vi "read allowed execution modes.vi"(8 "error in":errorcluster, 11 "Modbus Slave editor node in":refnum<class "Modbus Slave editor node.lvclass">) -> (0 "error out":errorcluster, 2 "allowed execution modes":T1[](array[typedef]), 3 "Modbus Slave editor node out":refnum<class "Modbus Slave editor node.lvclass">)   [LabVIEW 2013, in "Modbus Slave editor node.lvclass"]
doc: "Platypus Framework 1.0.1.65\nNI Systems Engineering - National Instruments"
uses:
  Modbus Slave editor node.lvclass
  <vilib>/NI/Tag Bus Data Framework/Configuration Editor/Classes/Module editor node/Allowed Execution Modes.ctl
  <vilib>/NI/Tag Bus Data Framework/Configuration Editor/Classes/Module editor node/module editor node.lvclass
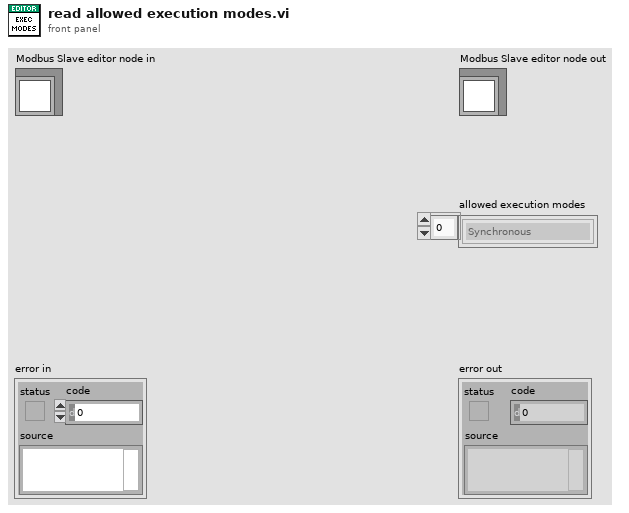
[diagram p1: front panel]
types:
  T1 = typedef "PL Framework Configuration Tool.lvlib/module editor node.lvclass/Allowed Execution Modes.ctl" = enum16{"Synchronous", "Asynchronous"}
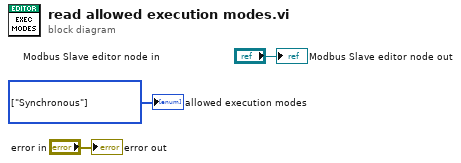
[diagram p0: block diagram]
diagram:
  w1 = T1[] [enum."Synchronous"] items=["Synchronous", "Asynchronous"] ("allowed execution modes")
  "error out" <- "error in"
  "Modbus Slave editor node out" <- "Modbus Slave editor node in"
  "allowed execution modes" <- w1
